vi "test Set All Endpoint Configurations Updates Possible Connections.vi"(8 "error in (no error)":errorcluster, 11 "TestCase in":refnum<class "SLSC Switch Scripting Unit Tests.lvclass">) -> (0 "error out":errorcluster, 3 "TestCase out":refnum<class "SLSC Switch Scripting Unit Tests.lvclass">)   [LabVIEW 2017, in "SLSC Switch Scripting Unit Tests.lvclass"]
uses:
  SLSC Switch Scripting Unit Tests.lvclass
  Properties/SLSC Switch All Properties.ctl
  Shared/Routing and Faulting Hardware API/Types/Possible Connections for Endpoint.ctl
  Shared/Endpoint Configuration Cluster.ctl
  Shared/Endpoint Configuration Enum.ctl
  SLSC Switch Scripting Unit Tests.lvclass/SLSC Switch Scripting Unit Tests.ctl
  Custom Device/Find All SLSC Switch Custom Devices.vi
  <vilib>/addons/_JKI Toolkits/VI Tester/TestCase.llb/TestCase.lvclass
  SLSC Switch Scripting.lvlib
  Shared/Routing and Faulting Hardware API/Routing and Faulting Hardware API.lvlib
  Shared/SLSC Switch Shared.lvlib
  C:/Program Files (x86)/National Instruments/LabVIEW 2017/vi.lib/addons/_JKI Toolkits/VI Tester/TestCase.llb/TestCase.lvclass
panel:
  in  "Save?":bool
  out "Output Filename":string
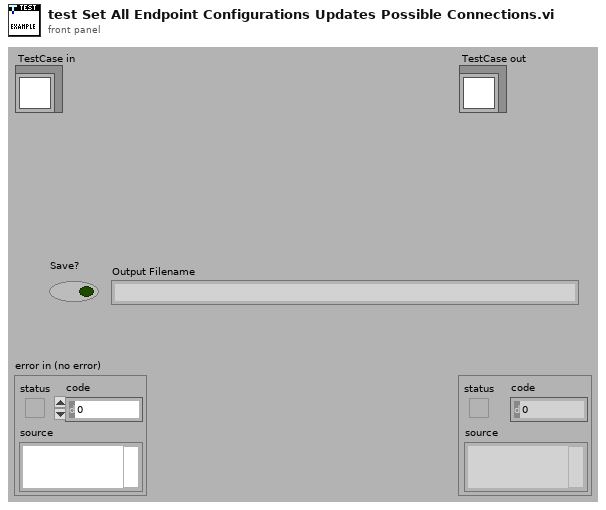
[diagram p1: front panel]
types:
  T1 = typedef "SLSC Switch Shared.lvlib/Endpoint Configuration Cluster.ctl" = cluster{"Endpoint":string, "Configuration":T2}
  T2 = typedef "SLSC Switch Shared.lvlib/Endpoint Configuration Enum.ctl" = enum16{"Load", "Source", "Configuration"}
  T3 = typedef "Routing and Faulting Hardware API.lvlib/Possible Connections for Endpoint.ctl" = cluster{"Source":string, "Destinations":string[]}
  T4 = typedef "SLSC Switch Scripting.lvlib/SLSC Switch All Properties.ctl" = cluster{"Model":string, "Resource":string, "Topology":string, "Capabilities":string, "Description":string}
  T5 = typedef "Custom Device API.lvlib/Custom Device Item Ref.ctl" = u64
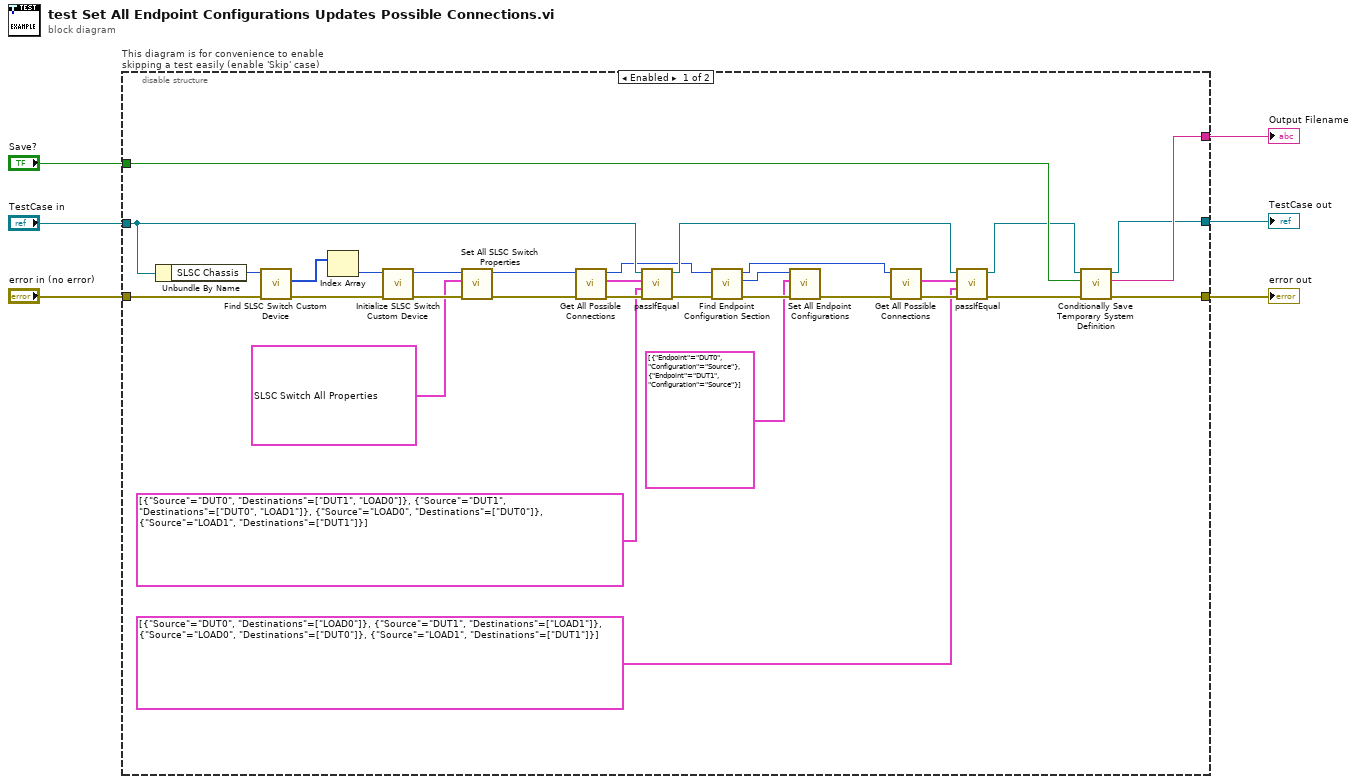
[diagram p0: block diagram]
diagram:
  n1 = disable-structure "This diagram is for convenience to enable skipping a test easily (enable 'Skip' case)" shown="Enabled" {
    disable-tunnel: "TestCase in" -> [w22 w41]
    disable-tunnel: [w35 w39] -> w3
    disable-tunnel: [w36 w40] -> w5
    disable-tunnel: "error in (no error)" -> [w29 w38]
    disable-tunnel: [w37 _] -> w2
    disable-tunnel: "Save?" -> [w34 _]
    frame Enabled {
      n2 = Unbundle By Name(w22) -> ("SLSC Chassis"=w30:u64)
      n3 = call-poly "Find SLSC Switch Custom Device.vi"("error in (no error)"=w29, "SLSC Chassis Ref"=w30) -> ("error out"=w32:errorcluster, "SLSC Switch Custom Device Ref IDs"=w33:T5[])  [unwired: 7 in, 1 out]
      n4 = Index Array(array=w33) -> (element=w31:T5)  [unwired: 1 in]
      n5 = call "Initialize SLSC Switch Custom Device.vi"("error in (no error)"=w32, "SLSC Switch Custom Device Ref in"=w31) -> ("error out"=w27:errorcluster, "SLSC Switch Custom Device Ref out"=w28:T5)  [unwired: 7 in, 1 out]
      n6 = call "Set All SLSC Switch Properties.vi"("error in (no error)"=w27, "SLSC Switch All Properties"=T4 {"Model"="Fake Device", "Resource"="SLSC-12001-0314B262-Mod4", "Topology"="SimpleTopology", "Capabilities"="{\n   \"switchesSpecVersion\": 1,\n   \"relays\": [\n      {\n         \"name\": \"DUT0_LOAD0\",\n         \"actions\": [\n            {\n               \"type\": \"property\",\n               \"resource\": \"Foo\",\n               \"value\": \"Vendor.DUT0_LOAD0\"\n            },\n            {\n               \"type\": \"command\",\n               \"resource\": \"Foo\",\n               \"value\": \"Vendor.Update\"\n            }\n         ]\n      },\n      {\n         \"name\": \"DUT1_LOAD1\",\n         \"actions\": [\n            {\n               \"type\": \"property\",\n               \"resource\": \"Foo\",\n               \"value\": \"Vendor.DUT1_LOAD1\"\n            },\n            {\n               \"type\": \"command\",\n               \"resource\": \"Foo\",\n               \"value\": \"Vendor.Update\"\n            }\n         ]\n      },\n      {\n         \"name\": \"DUT0_DUT1\",\n         \"actions\": [\n            {\n               \"type\": \"property\",\n               \"resource\": \"Foo\",\n               \"value\": \"Vendor.DUT0_DUT1\"\n            },\n            {\n               \"type\": \"command\",\n               \"resource\": \"Foo\",\n               \"value\": \"Vendor.Update\"\n            }\n         ]\n      }\n   ],\n   \"topologies\": [\n      {\n         \"name\": \"SimpleTopology\",\n         \"initialState\": {\n            \"open\": [\n               \"DUT0_LOAD0\",\n               \"DUT1_LOAD1\",\n               \"DUT0_DUT1\"\n            ],\n            \"close\": []\n         },\n         \"channelList\": {\n            \"names\": [\n               \"DUT0\",\n               \"DUT1\",\n               \"LOAD0\",\n               \"LOAD1\"\n            ]\n         },\n         \"connectionList\": [\n            {\n               \"src\": \"DUT0\",\n               \"dest\": \"LOAD0\",\n               \"relays\": [\n                  \"DUT0_LOAD0\"\n               ]\n            },\n            {\n               \"src\": \"DUT1\",\n               \"dest\": \"LOAD1\",\n               \"relays\": [\n                  \"DUT1_LOAD1\"\n               ]\n            },\n            {\n               \"src\": \"DUT0\",\n               \"dest\": \"DUT1\",\n               \"relays\": [\n                  \"DUT0_DUT1\"\n               ]\n            }\n         ]\n      },\n      {\n         \"name\": \"EvenSimplerTopology\",\n         \"initialState\": {\n            \"open\": [\n               \"DUT0_LOAD0\",\n               \"DUT1_LOAD1\"\n            ],\n            \"close\": []\n         },\n         \"channelList\": {\n            \"names\": [\n               \"DUT0\",\n               \"DUT1\",\n               \"LOAD0\",\n               \"LOAD1\"\n            ]\n         },\n         \"connectionList\": [\n            {\n               \"src\": \"DUT0\",\n               \"dest\": \"LOAD0\",\n               \"relays\": [\n                  \"DUT0_LOAD0\"\n               ]\n            },\n            {\n               \"src\": \"DUT1\",\n               \"dest\": \"LOAD1\",\n               \"relays\": [\n                  \"DUT1_LOAD1\"\n               ]\n            }\n         ]\n      }\n   ],\n   \"multiStateRelays\": []\n}", "Description"=""}, "SLSC Switch Custom Device Ref in"=w28) -> ("error out"=w25:errorcluster, "SLSC Switch Custom Device Ref out"=w24:T5)  [unwired: 7 in]
      n7 = call "Get All Possible Connections.vi"("error in (no error)"=w25, "Hardware Ref in"=w24) -> ("error out"=w23:errorcluster, "Possible Connections"=w19:T3[], "Hardware Ref out"=w10:T5)  [unwired: 7 in]
      n8 = call-dynamic "passIfEqual.vi"("error in (no error)"=w23, "y"=T3[] [{"Source"="DUT0", "Destinations"=["DUT1", "LOAD0"]}, {"Source"="DUT1", "Destinations"=["DUT0", "LOAD1"]}, {"Source"="LOAD0", "Destinations"=["DUT0"]}, {"Source"="LOAD1", "Destinations"=["DUT1"]}] ("Possible Connections"), "x"=w19, "TestCase in"=w22) -> ("error out"=w21:errorcluster, "TestCase out"=w15:refnum<class "SLSC Switch Scripting Unit Tests.lvclass">)  [unwired: 6 in]
      n9 = call "Find Endpoint Configuration Section.vi"("error in (no error)"=w21, "SLSC Switch Custom Device Ref in"=w10) -> ("error out"=w11:errorcluster, "Endpoint Config Section Ref"=w9:T5, "SLSC Switch Custom Device Ref out"=w8:T5)  [unwired: 7 in]
      n10 = call "Set All Endpoint Configurations.vi"("error in (no error)"=w11, "All Endpoint Configurations"=T1[] [{"Endpoint"="DUT0", "Configuration"=enum."Source"}, {"Endpoint"="DUT1", "Configuration"=enum."Source"}], "Endpoint Configuration Section Ref in"=w9) -> ("error out"=w16:errorcluster)  [unwired: 7 in, 1 out]
      n11 = call "Get All Possible Connections.vi"("error in (no error)"=w16, "Hardware Ref in"=w8) -> ("error out"=w18:errorcluster, "Possible Connections"=w17:T3[])  [unwired: 7 in, 1 out]
      n12 = call-dynamic "passIfEqual.vi"("error in (no error)"=w18, "y"=T3[] [{"Source"="DUT0", "Destinations"=["LOAD0"]}, {"Source"="DUT1", "Destinations"=["LOAD1"]}, {"Source"="LOAD0", "Destinations"=["DUT0"]}, {"Source"="LOAD1", "Destinations"=["DUT1"]}] ("Possible Connections"), "x"=w17, "TestCase in"=w15) -> ("error out"=w13:errorcluster, "TestCase out"=w14:refnum<class "SLSC Switch Scripting Unit Tests.lvclass">)  [unwired: 6 in]
      n13 = call "Conditionally Save Temporary System Definition.vi"("error in (no error)"=w13, "Save?"=w34, "Test Case"=w14) -> ("error out"=w36:errorcluster, "filename"=w37:string, "Test Case"=w35:refnum<class "SLSC Switch Scripting Unit Tests.lvclass">)  [unwired: 6 in]
    }
    frame Disabled {
      # "skip test result while test is under development"
      n14 = call <vilib>:"skip.vi"("error in (no error)"=w38, "TestCase in"=w41) -> ("error out"=w40:errorcluster, "TestCase out"=w39:refnum<class "SLSC Switch Scripting Unit Tests.lvclass">)  [unwired: 8 in]
    }
  }
  "error out" <- w5
  "TestCase out" <- w3
  "Output Filename" <- w2
